vi "Create NET REST Client.vi"(5 "REST Client_NET in":refnum<class "REST Client_NET.lvclass">, 6 "Default Headers ([JSON])":T1[](array[typedef])=[{"header"="Content-Type", "value"="application/json"}], 7 "LabVIEWHTTPClient_NET":refnum<class "LabVIEWHTTPClient_NET.lvclass">, 8 "error in (no error)":errorcluster, 10 "Escape URLs (true)":bool=TRUE, 11 "Base URL":string) -> (0 "error out":errorcluster, 3 "REST Client_NET out":refnum<class "REST Client_NET.lvclass">)   [LabVIEW 2018, in "REST Client_NET.lvlib" / "REST Client_NET.lvclass"]
uses:
  REST Client_NET.lvclass
  C:/Program Files (x86)/National Instruments/LabVIEW 2018/vi.lib/addons/_JKI.lib/REST Client/classes/REST Client/REST Client.lvclass
  <vilib>/addons/_JKI.lib/REST Client/classes/REST Client/HTTP Header.ctl
  LabVIEWHTTPClient_NET/LabVIEWHTTPClient_NET.lvclass
  REST Client_NET.lvclass/REST Client_NET.ctl
  <vilib>/addons/_JKI.lib/REST Client/classes/REST Client/REST Client.lvclass
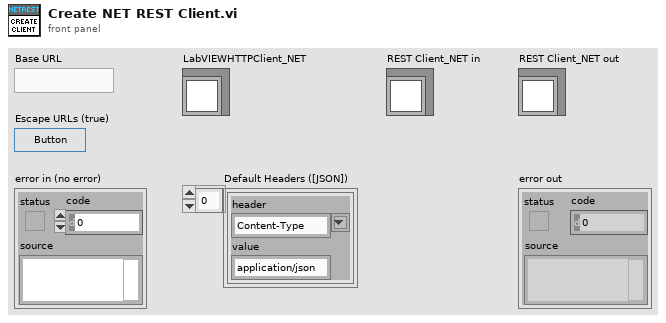
[diagram p1: front panel]
types:
  T1 = typedef "REST Client.lvlib/REST Client.lvclass/HTTP Header.ctl" = cluster{"header":string, "value":string}
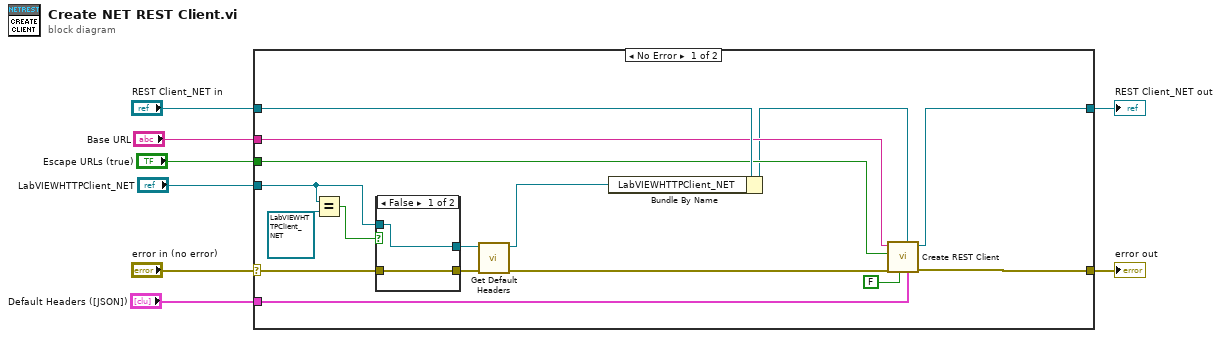
[diagram p0: block diagram]
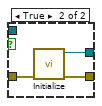
[diagram p2: hidden frame]
diagram:
  n1 = case shown="No Error" "error in (no error)" {
    selector: "error in (no error)" -> [w17 w31]
    tunnel: [w22 w31] -> w7
    tunnel: [w23 w30] -> w5
    tunnel: "REST Client_NET in" -> [w24 w30]
    tunnel: "Default Headers ([JSON])" -> [w10 _]
    tunnel: "Base URL" -> [w21 _]
    tunnel: "Escape URLs (true)" -> [w20 _]
    tunnel: "LabVIEWHTTPClient_NET" -> [w15 _]
    frame No Error {
      n2 = Equal?(x=w15, y=refnum<class "LabVIEWHTTPClient_NET.lvclass"> refnum) -> (x = y?=w16:bool)
      n3 = case shown="False" w16 {
        tunnel: w17 -> [w25 w29]
        tunnel: [w25 w28] -> w14
        tunnel: [w26 w27] -> w13
        tunnel: w15 -> [w26 _]
        frame False {
        }
        frame True {
          n4 = call "Initialize.vi"("error in (no error)"=w29) -> ("error out"=w28:errorcluster, "HTTP Client Out"=w27:refnum<class "LabVIEWHTTPClient_NET.lvclass">)  [unwired: 9 in]
        }
      }
      n5 = call "Get Default Headers.vi"("error in (no error)"=w14, "LabVIEWHTTPClient_NET in"=w13) -> ("error out"=w12:errorcluster, "LabVIEWHTTPClient_NET out"=w11:refnum<class "LabVIEWHTTPClient_NET.lvclass">)  [unwired: 7 in, 1 out]
      n6 = Bundle By Name(cluster=w24, "LabVIEWHTTPClient_NET"=w11) -> (w19:refnum<class "REST Client_NET.lvclass">)
      n7 = call <vilib>:"Create REST Client.vi"("Default Headers ([JSON])"=w10, "REST Client in"=w19, "Verify Server(true)"=FALSE, "error in (no error)"=w12, "Escape URLs (true)"=w20, "Base URL"=w21) -> ("error out"=w22:errorcluster, "REST Client out"=w23:refnum<class "REST Client_NET.lvclass">)  [unwired: 4 in]
    }
    frame Error {
    }
  }
  "error out" <- w7
  "REST Client_NET out" <- w5
